vi "NDMotor_MvBkwTest.vi"() -> ()   [LabVIEW 2024]
panel:
  out "move time (ms)":i32
  out "steps":i32
  out "error out":errorcluster
  out "VISA resource name out":refnum<visa-resource-name>
  in  "error in":errorcluster
  in  "VISA resource name":refnum<visa-resource-name>
  in  "Steps":i32
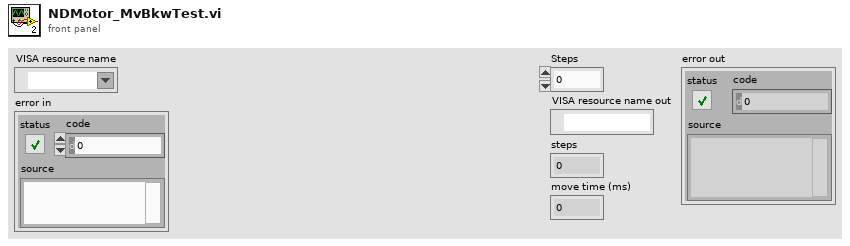
[diagram p1: front panel]
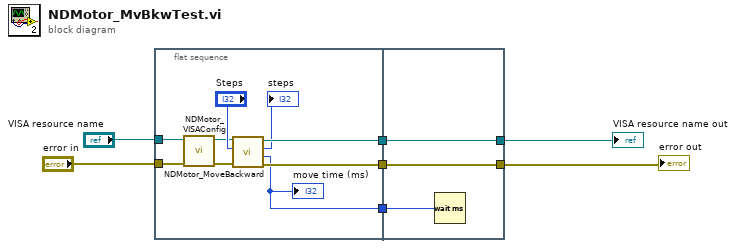
[diagram p0: block diagram]
diagram:
  n1 = flat-sequence {
    tunnel: "VISA resource name" -> [w13]
    tunnel: "error in" -> [w12]
    tunnel: [w8] -> w5
    tunnel: [w11] -> w4
    tunnel: [w10] -> w2
    tunnel: w5 -> [w19]
    tunnel: w4 -> [w18]
    tunnel: [w18] -> w3
    tunnel: w2 -> [w17]
    tunnel: [w17] -> w1
    frame #0 {
      n2 = call "NDMotor_VISAConfig.vi"("error in"=w12, "VISA resource name"=w13) -> ("error out"=w14:errorcluster, "reference out"=w15:refnum<visa-resource-name>)  [unwired: 8 in]
      n3 = call "NDMotor_MoveBackward.vi"("error in"=w14, "Steps"="Steps", "VISA resource name"=w15) -> ("error out"=w10:errorcluster, "move time (ms)"=w8:i32, "steps"=→"steps":i32, "VISA resource name out"=w11:refnum<visa-resource-name>)  [unwired: 5 in]
      "move time (ms)" <- w8
    }
    frame #1 {
      n4 = Wait (ms)(milliseconds to wait=w19) -> ()  [unwired: 1 out]
    }
  }
  "VISA resource name out" <- w3
  "error out" <- w1
